vi "Process.vi"(8 "error in":errorcluster, 11 "DAQ_Manager":refnum<class "DAQ_Manager.lvclass">) -> (0 "error out":errorcluster, 3 "DAQ_Manager out":refnum<class "DAQ_Manager.lvclass">)   [LabVIEW 2019, in "DAQ_Manager.lvclass"]
doc: "---------------------------------------------------------------\nJKI State Machine Objects™\nhttp://jki.net/state-machine-objects/\nCopyright (C) 2005-2015, JKI <info@jki.net>\nALL RIGHTS RESERVED"
uses:
  DAQ_Manager.lvclass
  <vilib>/JKI/JKI SMO/SMO/SMO.lvclass
  <vilib>/JKI/JKI SMO/SMO/Typedefs/Parent Call--Enum.ctl
  DAQ/DAQ.lvclass
  DAQ/Typedefs/PublicEvents--DAQ.Read.ctl
  DAQ/Typedefs/PublicEvents--DAQ.Write.ctl
  DAQ/Typedefs/PrivateEvents--DAQ.AI.Channels.ctl
  DAQ/Typedefs/DAQ_Type.ctl
  DAQ/Typedefs/DAQ_SamplingInfo.ctl
  DAQ/Typedefs/DAQ_SamplingMode.ctl
  DAQ/Typedefs/DAQ_Config.ctl
  DAQmx.AO/Typedefs/DAQmx.AO_Config.ctl
  DAQmx.AI/Typedefs/DAQmx.AI_Config.ctl
  DAQmx.AI/Typedefs/AI.Terminal-enum.ctl
  DAQmx.AI/Typedefs/AI.Coupling-enum.ctl
  DAQmx.AO/Typedefs/AO.Terminal-enum.ctl
  Typedefs/PrivateEvents--DAQ_Manager.setDAQConfig.ctl
  C:/Program Files (x86)/National Instruments/LabVIEW 2016/vi.lib/JKI/JKI SMO/SMO/SMO.lvclass
  DAQmx.AI/DAQmx.AI.lvclass
  F:/user/patrick/levy_inst_lockin/src/SMOs/DAQmx/DAQmx.lvclass
  DAQmx.AO/DAQmx.AO.lvclass
  DAQmx/DAQmx.lvclass
  F:/user/patrick/levy_inst_lockin/src/SMOs/DAQ/DAQ.lvclass
  <vilib>/JKI/JKI SMO/SMO/Typedefs/SMOState --Enum.ctl
panel:
  out "DAQ.Read (ms)":u32
  out "DAQ.Read Aggregate (ms)":u32
  out "setWaveform (ms)":u32
  out "Array 2":string[](array[string])
  out "Array":T1[](array[typedef])
  in  "Update Config?":bool
  in  "DAQmx.AO.config":T2[](array[typedef])=[{"output terminal configuration"=-1}] {"output terminal configuration" items=["Default"=-1, "RSE"=10083, "Differential"=10106, "Pseudodifferential"=12529]}
  in  "DAQmx.AI.config":T4[](array[typedef])=[{"AI.Coupling"=10045, "input terminal configuration "=-1}] {"input terminal configuration" items=["default"=-1, "RSE"=10083, "NRSE"=10078, "Differential"=10106, "Pseudodifferential"=12529]; "AI.Coupling" items=["AC"=10045, "DC"=10050, "GND"=10066]}
  in  "DAQ.Config (AO)":T7[](array[typedef])=[{"Channels"="PXI1Slot2/ao0", "DAQ_Type"=enum."AO", "minimum value"=-10.0, "maximum value"=10.0, "DAQ_SamplingInfo"={"Fs"=1000.0, "#s"=1000}, "DAQ_SamplingMode"=enum."Continuous"}] {"maximum value" format="%0.2f"; "minimum value" format="%0.2f"}
  in  "DAQ.Config (AI)":T7[](array[typedef])=[{"Channels"="PXI1Slot2/ai0", "DAQ_Type"=enum."AI", "minimum value"=-10.0, "maximum value"=10.0, "DAQ_SamplingInfo"={"Fs"=1000.0, "#s"=1000}, "DAQ_SamplingMode"=enum."Continuous"}] {"maximum value" format="%0.2f"; "minimum value" format="%0.2f"}
  in  "DAQmx Physical Channels (AO)":tag="PXI1Slot2/ao0:1, PXI1Slot3/ao0:1, PXI1Slot4/ao0:1, PXI1Slot5/ao0:1"
  in  "DAQmx Physical Channels (AI)":tag="PXI1Slot2/ai0:1, PXI1Slot3/ai0:1, PXI1Slot4/ai0:1, PXI1Slot5/ai0:1"
  in  "Simulate?":bool
  # "1. Make a lot of these controls hidden on default Main UI\n    (eg, output terminal)\n2. DAQ.Config etc should be arrays, with each element per device\n3. Make use of most recent lockin controls on front panel\n-- use new enums and arrays per channel/device\n4. DAQ_Manager needs an API for setting the DAQ config (setConfig?)\n5. In process.vi if any Config settings are changed: go to:\nDAQ: stop SMO\nDAQ: init\nDAQ: start SMO\n6. I don't think these need to be controls here in process.vi, they can just be\nchanged through public methods."
  # "DAQ Manager Process.vi"
  # "For instructions on how to use the JKI State Machine Objects, examples and video tutorials, visit:\nhttp://jki.net/state-machine-objects/\n\nJKI State Machine Objects™\nhttp://jki.net/state-machine-objects/\nCopyright (C) 2005-2015, JKI <info@jki.net>\nALL RIGHTS RESERVED"
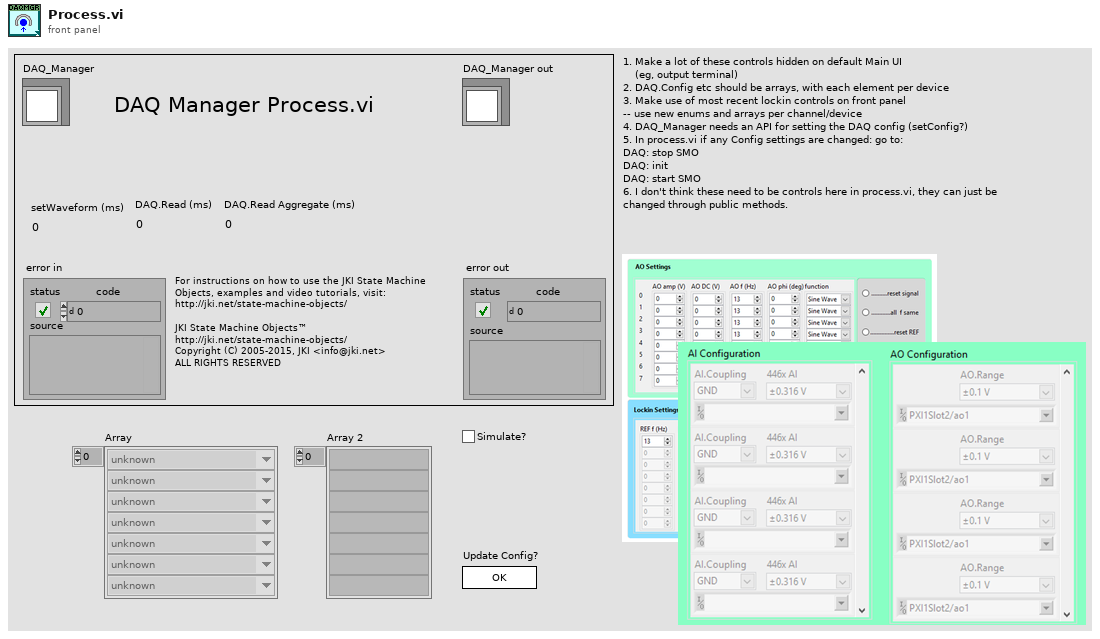
[diagram p1: front panel]
types:
  T1 = typedef "SMO.lvclass/SMOState --Enum.ctl" = enum16{"unknown", "Created", "Started", "Stopped"}
  T2 = typedef "DAQmx.AO.lvclass/DAQmx.AO_Config.ctl" = cluster{"output terminal configuration":T3}
  T3 = typedef "DAQmx.AO.lvclass/AO.Terminal-enum.ctl" = i32
  T4 = typedef "DAQmx.AI.lvclass/DAQmx.AI_Config.ctl" = cluster{"AI.Coupling":T5, "input terminal configuration ":T6}
  T5 = typedef "DAQmx.AI.lvclass/AI.Coupling-enum.ctl" = i32
  T6 = typedef "DAQmx.AI.lvclass/AI.Terminal-enum.ctl" = i32
  T7 = typedef "DAQ.lvclass/DAQ_Config.ctl" = cluster{"Channels":T8, "DAQ_Type":T9, "minimum value":dbl, "maximum value":dbl, "DAQ_SamplingInfo":T10, "DAQ_SamplingMode":T11}
  T8 = typedef "DAQ.lvclass/PrivateEvents--DAQ.AI.Channels.ctl" = string
  T9 = typedef "DAQ.lvclass/DAQ_Type.ctl" = enum16{"AI", "AO"}
  T10 = typedef "DAQ.lvclass/DAQ_SamplingInfo.ctl" = cluster{"Fs":dbl, "#s":i32}
  T11 = typedef "DAQ.lvclass/DAQ_SamplingMode.ctl" = enum16{"Continuous", "Finite"}
  T12 = typedef "SMO.lvclass/Parent Call--Enum.ctl" = enum16{"Allows parent to run", "Does not request parent to run"}
  T13 = typedef "DAQ_Manager.lvclass/PrivateEvents--DAQ_Manager.setDAQConfig.ctl" = cluster{"DAQ.Config (AI)":cluster{"Channels":string, "DAQ_Type":enum16{"AI", "AO"}, "minimum value":dbl, "maximum value":dbl, "DAQ_SamplingInfo":cluster{"Fs":dbl, "#s":i32}, "DAQ_SamplingMode":enum16{"Continuous", "Finite"}}[], "DAQmx.AI.config":T4[], "DAQ.Config (AO)":cluster{"Channels":string, "DAQ_Type":enum16{"AI", "AO"}, "minimum value":dbl, "maximum value":dbl, "DAQ_SamplingInfo":cluster{"Fs":dbl, "#s":i32}, "DAQ_SamplingMode":enum16{"Continuous", "Finite"}}[], "DAQmx.AO.config":T2[]}
  T14 = enum32{"invalid app kind", "Development System", "Run Time System", "Student Edition", "Embedded LabVIEW", "Evaluation", "Custom"}
  T15 = enum32{"Invalid", "Standard", "Closed", "Hidden", "Minimized", "Maximized"}
  T16 = enum32{"Bad", "Idle", "Run top level", "Running"}
  T17 = typedef "DAQ.lvclass/PublicEvents--DAQ.Read.ctl" = waveform(dbl)[]
  T18 = cluster{"Core":cluster{"Current VI Reference":refnum<vi>, "Close Panel on Exit?":bool, "error":errorcluster}, "Self Reference":refnum<class "DAQ_Manager.lvclass">, "Your string data":string, "DAQ":refnum<class "DAQ.lvclass">[], "setWaveform":T17, "to":i32, "AI events":refnum<user-event>[], "DAQ.Config (AO)":T7[], "DAQ.Config (AI)":T7[], "DAQmx.AO.Config":T2[], "DAQmx.AI.Config":T4[]}
  T19 = cluster{"Channels":string, "DAQ_Type":enum16{"AI", "AO"}, "minimum value":dbl, "maximum value":dbl, "DAQ_SamplingInfo":cluster{"Fs":dbl, "#s":i32}, "DAQ_SamplingMode":enum16{"Continuous", "Finite"}}[]
  T20 = typedef "DAQ_Manager.lvclass/PrivateEvents--DAQ_Manager.setWaveform.ctl" = waveform(dbl)[]
  T21 = cluster{"Current VI Reference":refnum<vi>, "Close Panel on Exit?":bool, "error":errorcluster}
  T22 = typedef "SMO.lvclass/Protected Events.ctl" = cluster{"StopProcesses":refnum<user-event>, "AbortProcesses":refnum<user-event>, "Config Changed":refnum<user-event>, "Dependency":refnum<user-event>}
  T23 = typedef "DAQ_Manager.lvclass/PrivateEvents--Cluster.ctl" = cluster{"setWaveform":refnum<user-event>, "setDAQConfig":refnum<user-event>}
  T24 = typedef "DAQ_Manager.lvclass/PublicEvents--Cluster.ctl" = cluster{"getWaveform":refnum<user-event>}
  T25 = typedef "DAQ.lvclass/PublicEvents--Cluster.ctl" = cluster{"DAQ.Read":refnum<user-event>, "DAQ.Write":refnum<user-event>}
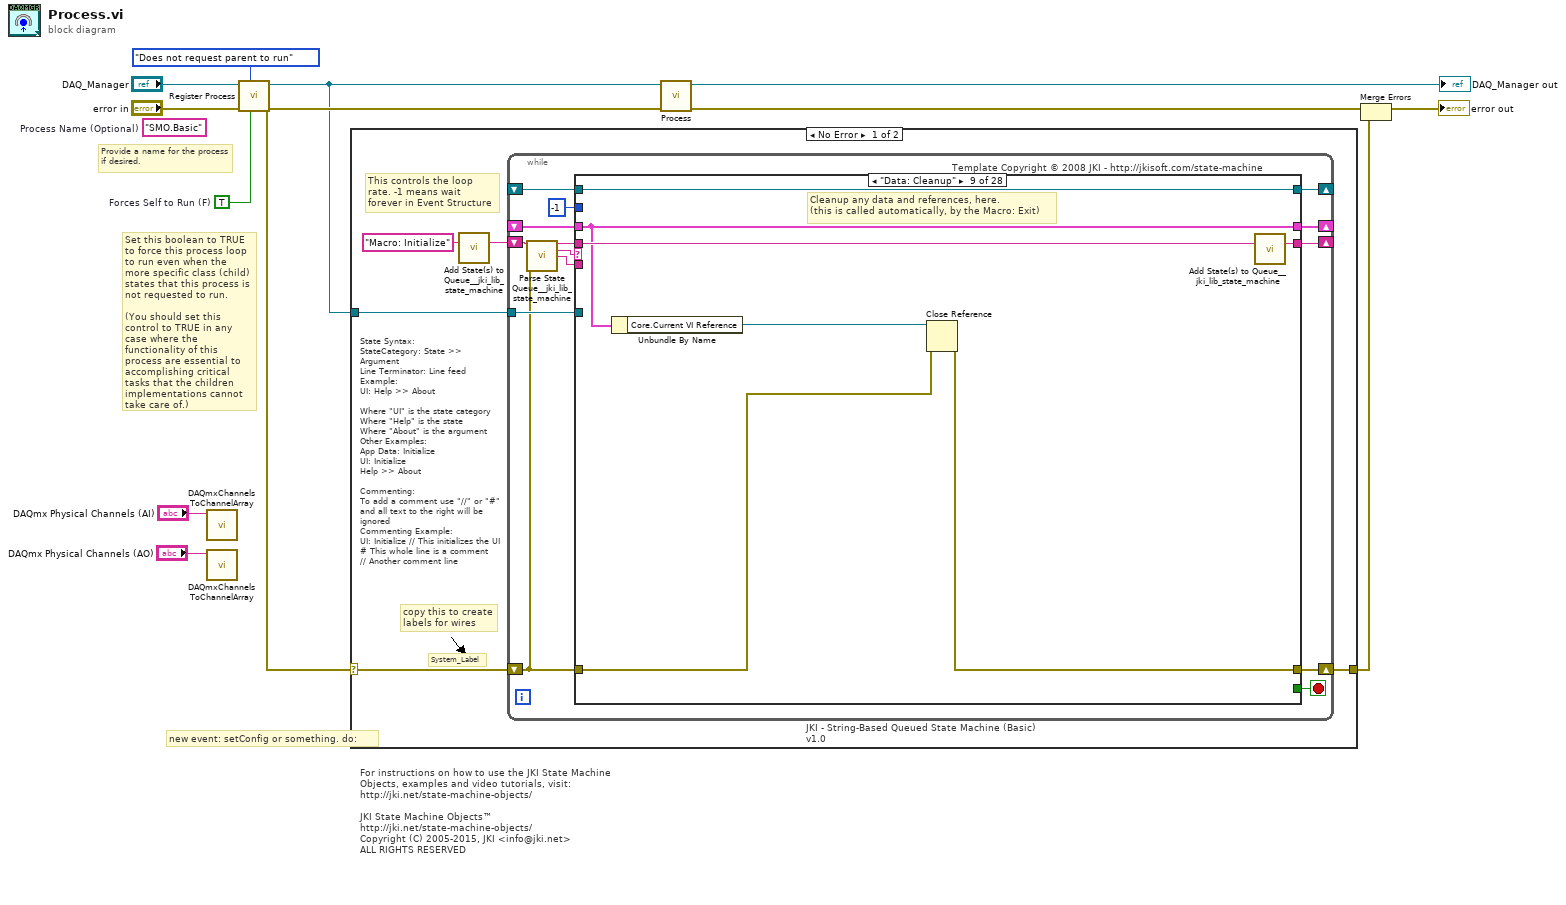
[diagram p0: block diagram]
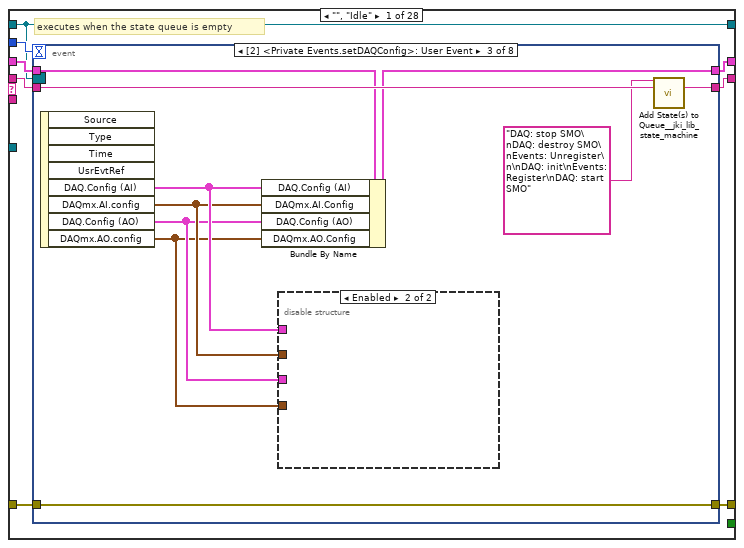
[diagram p2: hidden frame]
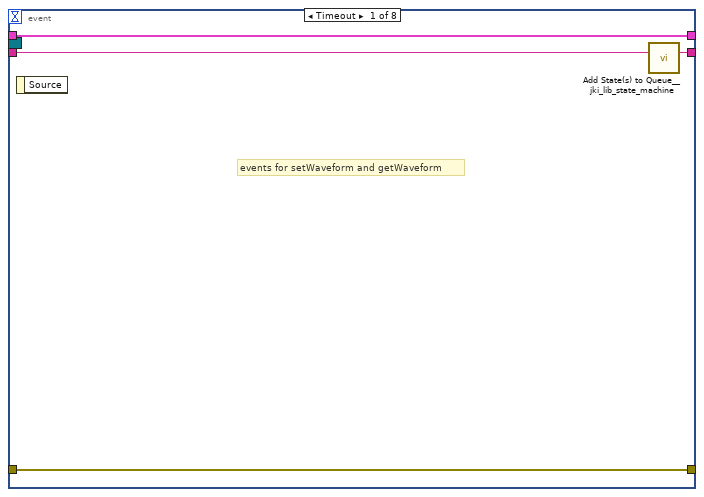
[diagram p3: hidden frame]
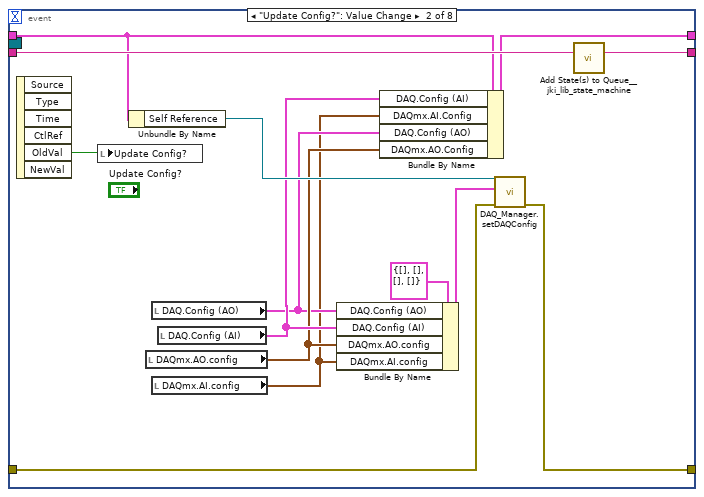
[diagram p4: hidden frame]
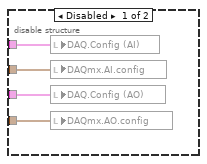
[diagram p5: hidden frame]
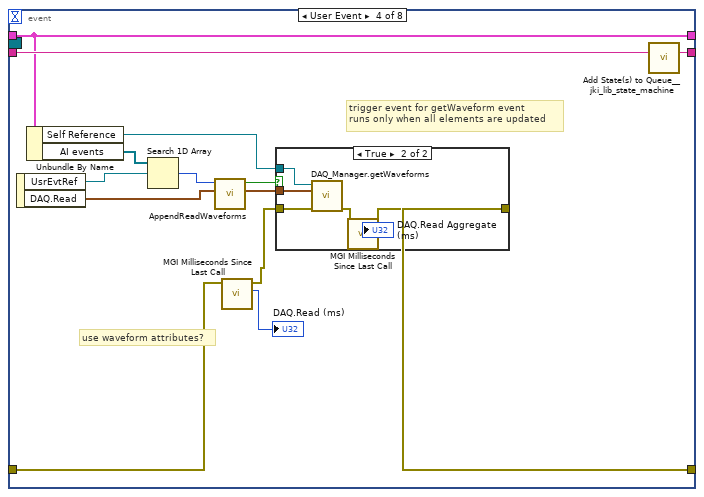
[diagram p6: hidden frame]
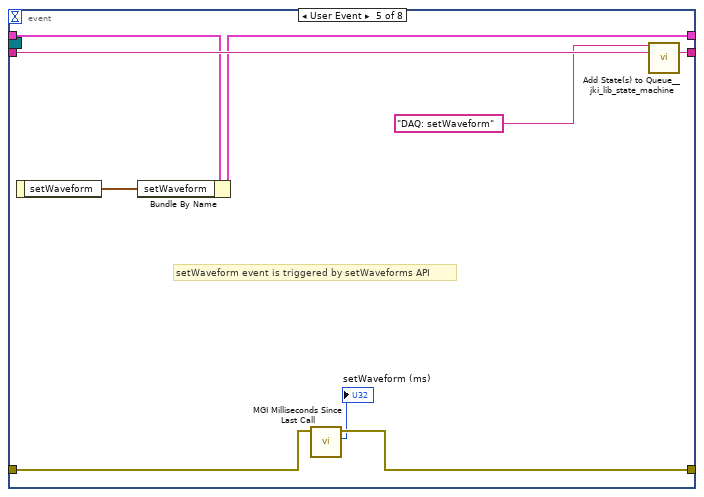
[diagram p8: hidden frame]
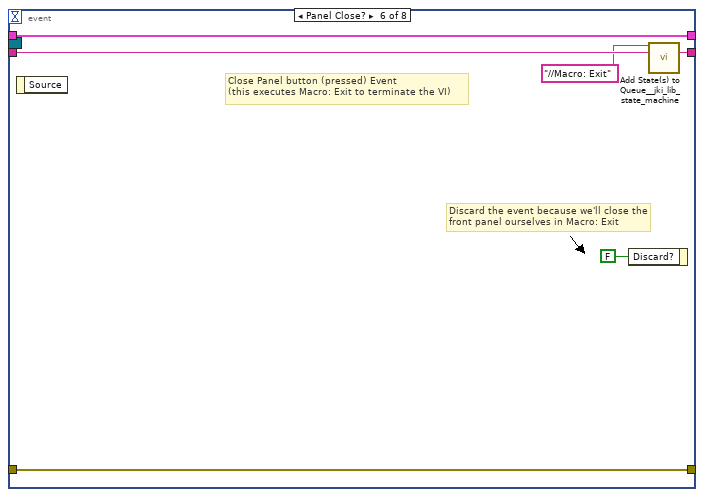
[diagram p9: hidden frame]
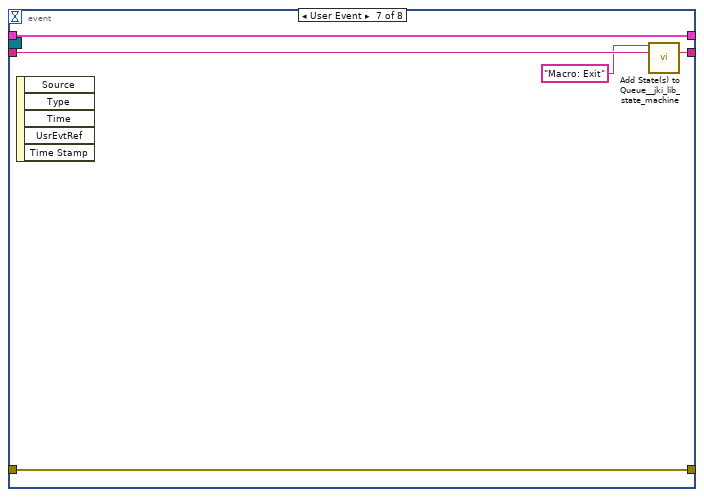
[diagram p10: hidden frame]
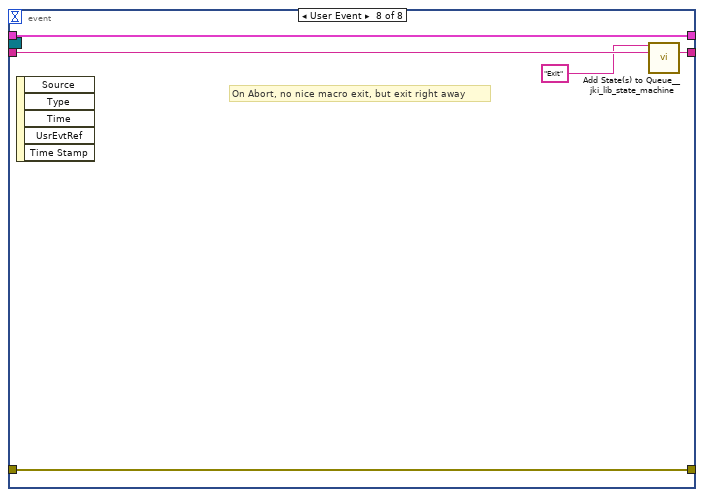
[diagram p11: hidden frame]
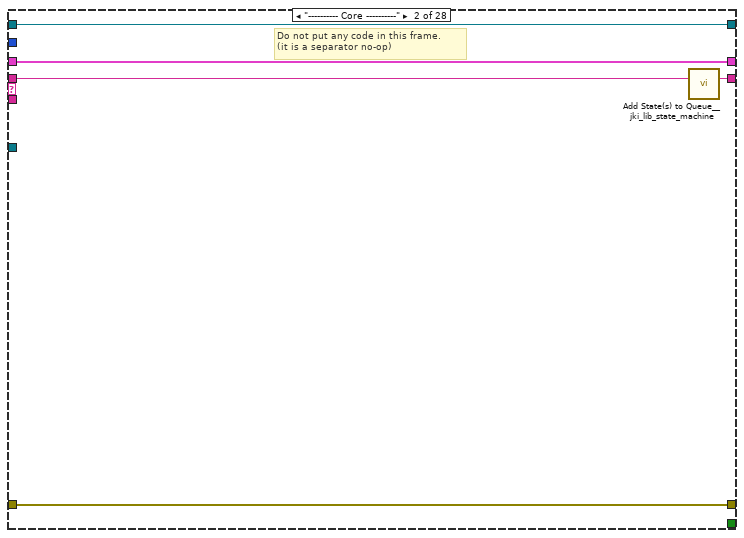
[diagram p12: hidden frame]
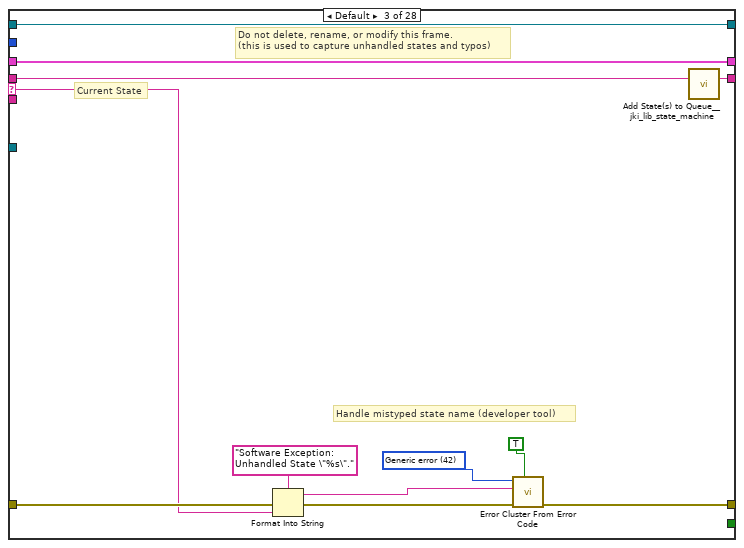
[diagram p13: hidden frame]
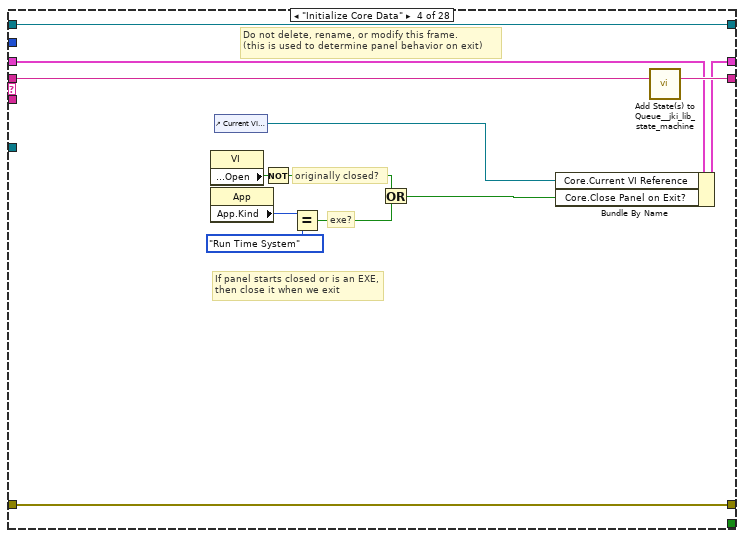
[diagram p14: hidden frame]
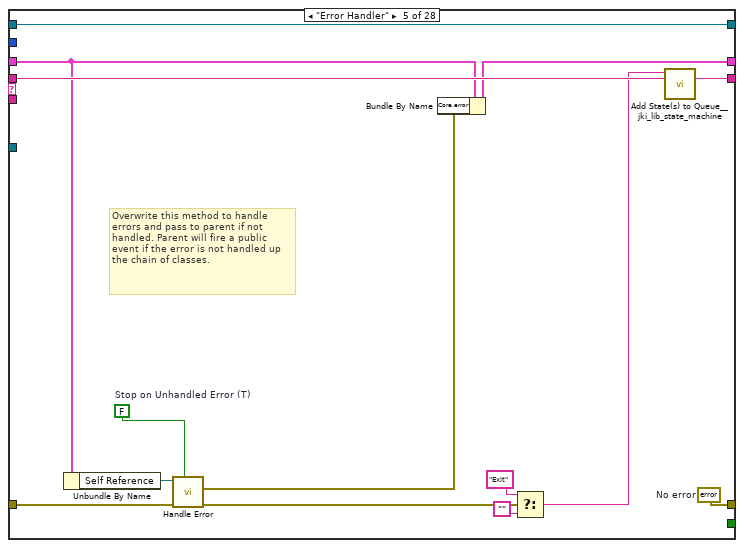
[diagram p15: hidden frame]
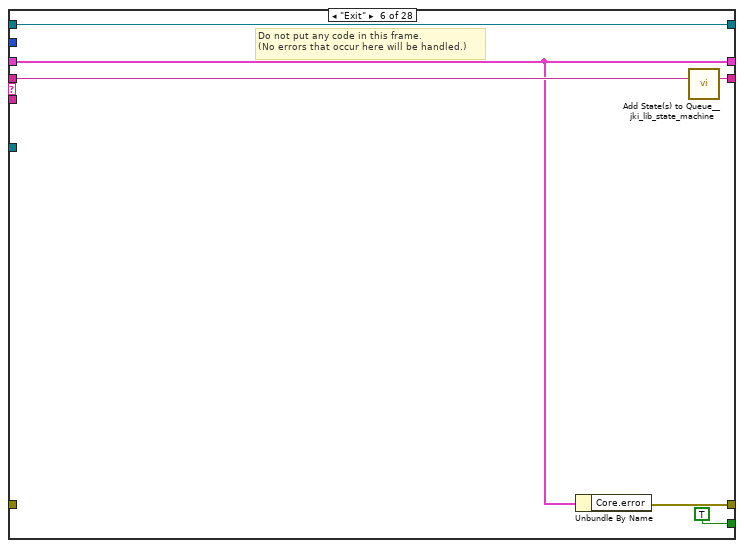
[diagram p16: hidden frame]
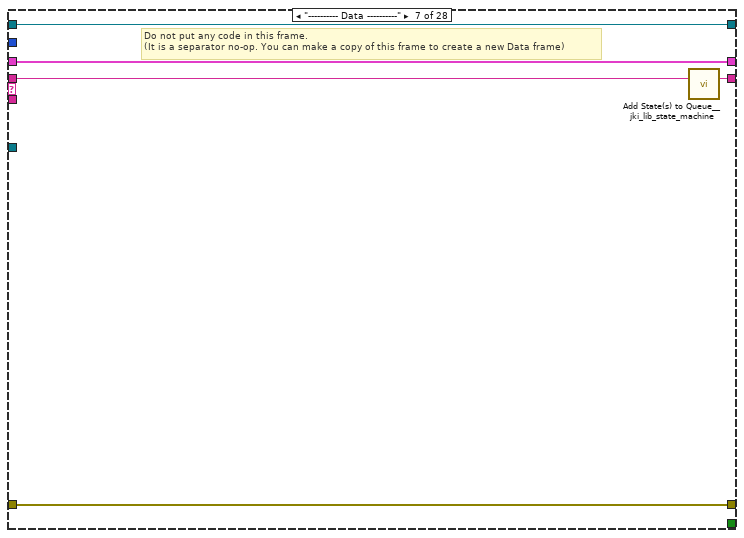
[diagram p17: hidden frame]
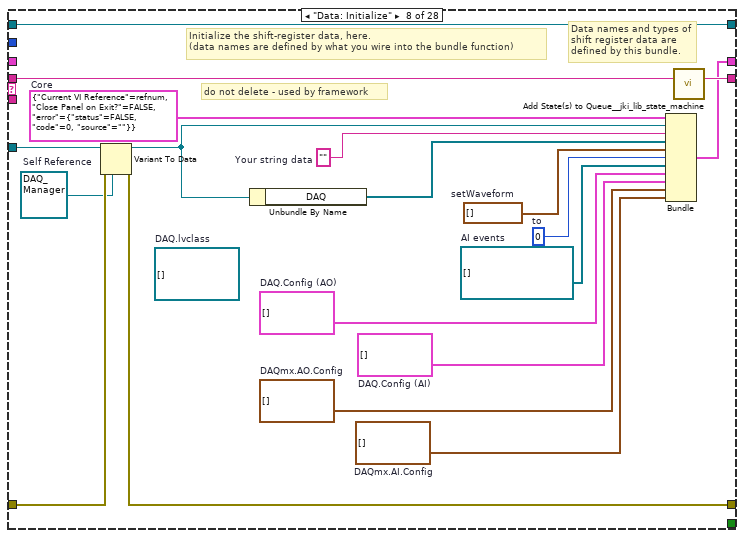
[diagram p18: hidden frame]
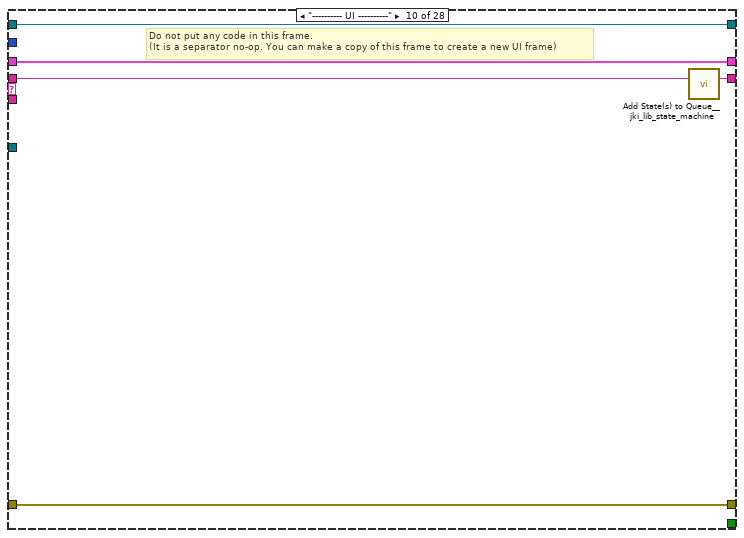
[diagram p19: hidden frame]
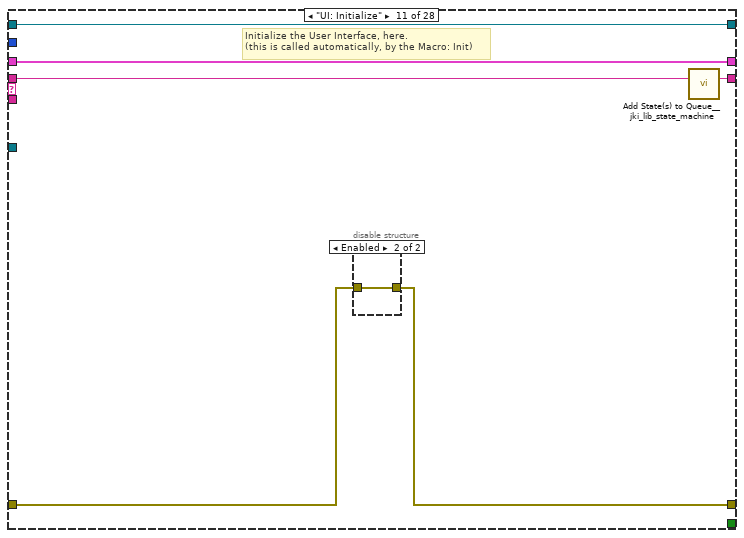
[diagram p20: hidden frame]
diagram:
  w3 = TRUE  # Forces Self to Run (F)
  (unwired) "SMO.Basic"  # Process Name (Optional)
  # "new event: setConfig or something. do:"
  # "Provide a name for the process\nif desired."
  # "Set this boolean to TRUE to force this process loop to run even when the more specific class (child) states that this process is not requested to run.\n\n(You should set this control to TRUE in any case where the functionality of this process are essential to accomplishing critical tasks that the children implementations cannot take care of.)"
  # "For instructions on how to use the JKI State Machine Objects, examples and video tutorials, visit:\nhttp://jki.net/state-machine-objects/\n\nJKI State Machine Objects™\nhttp://jki.net/state-machine-objects/\nCopyright (C) 2005-2015, JKI <info@jki.net>\nALL RIGHTS RESERVED"
  n1 = call "DAQmxChannelsToChannelArray.vi"("DAQmx Physical Channel"="DAQmx Physical Channels (AI)") -> ()  [unwired: 10 in, 1 out]
  n2 = call "DAQmxChannelsToChannelArray.vi"("DAQmx Physical Channel"="DAQmx Physical Channels (AO)") -> ()  [unwired: 10 in, 1 out]
  n3 = call <vilib>:"Register Process.vi"("Forces Self to Run (F)"=w3, "Parent Call"=Parent_Call--Enum."Does not request parent to run", "error in (no error)"="error in", "SMO"="DAQ_Manager") -> ("error out"=w9:errorcluster, "SMO out"=w8:refnum<class "DAQ_Manager.lvclass">)  [unwired: 6 in]
  n4 = case shown="No Error" w9 {
    selector: w9 -> [w14 w492]
    tunnel: w8 -> [w15 _]
    tunnel: [w13 w492] -> w5
    frame No Error {
      # "State Syntax:\nStateCategory: State >> Argument\nLine Terminator: Line feed\nExample:\nUI: Help >> About\n\nWhere \"UI\" is the state category\nWhere \"Help\" is the state\nWhere \"About\" is the argument\nOther Examples:\nApp Data: Initialize\nUI: Initialize\nHelp >> About\n\nCommenting:\nTo add a comment use \"//\" or \"#\" and all text to the right will be ignored\nCommenting Example:\nUI: Initialize // This initializes the UI\n# This whole line is a comment\n// Another comment line"
      # "copy this to create labels for wires"
      # "This controls the loop rate. -1 means wait forever in Event Structure"
      # "System_Label"
      n5 = call <vilib>:"Add State(s) to Queue__jki_lib_state_machine.vi"("State(s) in (\"\")"="Macro: Initialize") -> ("States Out"=w17:string)  [unwired: 14 in]
      n6 = while "JKI - String-Based Queued State Machine (Basic) v1.0" {
        shift-right: [w25] -> _
        shift-left: _ -> [w20]
        shift-right: [w19] -> w13
        shift-left: w14 -> [w21]
        shift-right: [w27] -> _
        shift-left: w17 -> [w28]
        tunnel: w15 -> [w24]
        shift-right: [w23] -> _
        shift-left: _ -> [w22]
        stop <- w26 stop-if-true
        # "Template Copyright © 2008 JKI - http://jkisoft.com/state-machine"
        n7 = call <vilib>:"Parse State Queue__jki_lib_state_machine.vi"("State Queue"=w28, "Error In (no error)"=w21) -> ("Remaining States"=w30:string, "Current State"=w31:string, "Arguments"=w29:string)  [unwired: 11 in]
        n8 = case shown="\"Data: Cleanup\"" w31 {
          selector: w31 -> [_ _ w124 _ _ _ _ _ _ _ _ _ _ _ _ _ _ _ _ _ _ _ _ _ _ _ _ _]
          tunnel: w30 -> [w39 w122 w128 w147 w161 w167 w172 w191 w198 w203 w209 w219 w237 w269 w283 w298 w303 w314 w319 w340 w357 w362 w377 w432 w448 w462 w476 w491]
          tunnel: w29 -> [_ _ _ _ _ _ _ _ _ _ _ w213 w232 _ _ _ _ _ _ _ _ _ _ _ _ _ _ _]
          tunnel: w20 -> [w37 w119 w126 w138 w155 w163 w169 _ w194 w200 w206 w217 w234 w266 w279 w289 w300 w311 w316 w332 w355 w360 w366 w428 w445 w459 w473 w488]
          tunnel: [w38 w121 w127 w146 w160 w166 w171 w190 w197 w202 w208 w218 w236 w268 w282 w297 w302 w313 w318 w339 w356 w361 w376 w431 w447 w461 w475 w490] -> w27
          tunnel: [_ _ _ _ _ TRUE _ _ _ _ _ _ _ _ _ _ _ _ _ _ _ _ _ _ _ _ _ _] -> w26
          tunnel: [w34 w119 w126 w145 w154 w163 w169 w181 w194 w200 w206 w217 w234 w266 w279 w289 w300 w311 w316 w331 w355 w360 w374 w428 w445 w459 w473 w488] -> w25
          tunnel: -1 ("to") -> [w33 _ _ _ _ _ _ _ _ _ _ _ _ _ _ _ _ _ _ _ _ _ _ _ _ _ _ _]
          tunnel: w24 -> [_ _ _ _ _ _ _ w185 _ _ _ _ _ _ _ _ _ _ _ _ _ _ _ _ _ _ _ _]
          tunnel: [w32 w118 w123 w135 w159 w164 w168 w184 w193 w199 w207 w216 w231 w265 w280 w290 w299 w312 w315 w338 w354 w359 w375 w430 w446 w460 w477 w489] -> w23
          tunnel: w22 -> [w32 w118 w123 w135 w159 w164 w168 w184 w193 w199 w207 w216 w231 w265 w280 w290 w299 w312 w315 _ w354 w359 w375 w430 w446 w460 w477 w489]
          tunnel: w21 -> [w35 w120 w129 w144 w157 _ w170 w188 w192 w201 w205 w215 w235 w267 w281 w296 w301 w306 w317 w336 w353 w358 w367 w429 w440 w455 w474 w484]
          tunnel: [w36 w120 w130 w144 w156 w162 w170 w187 w195 w201 w204 w214 w229 w267 w281 w296 w301 w305 w317 w325 w353 w358 w368 w423 w443 w457 w474 w485] -> w19
          frame "", "Idle" {
            # "executes when the state queue is empty"
            n9 = event shown="[2] <Private Events.setDAQConfig>: User Event" {
              selector: w32 -> [_ _ _ _ _ _ _ _]
              dyn-events: _ -> [_ _ _ _ _ _ _ _]
              timeout: w33 -> [_ _ _ _ _ _ _ _]
              tunnel: w39 -> [w43 w56 w66 w85 w101 w107 w112 w117]
              tunnel: [w42 w57 w67 w84 w100 w106 w111 w116] -> w38
              tunnel: w37 -> [w41 w51 w63 w83 w98 w104 w109 w114]
              tunnel: [w40 w44 w64 w77 w94 w105 w110 w115] -> w36
              tunnel: w35 -> [w40 w45 w64 w74 w95 w105 w110 w115]
              tunnel: [w41 w50 w62 w83 w97 w104 w109 w114] -> w34
              event Timeout {
                # "events for setWaveform and getWaveform"
                n10 = event-data() -> ()  [unwired: 1 in, 1 out]
                n11 = call <vilib>:"Add State(s) to Queue__jki_lib_state_machine.vi"("State(s) in (\"\")"=w43) -> ("States Out"=w42:string)  [unwired: 14 in]
              }
              event "Update Config?": Value Change {
                n12 = event-data() -> ("OldVal"=w55:bool)  [unwired: 1 in, 5 out]
                n13 = local write "Update Config?"(w55) -> ()
                n14 = Unbundle By Name(w51) -> ("Self Reference"=w52:refnum<class "DAQ_Manager.lvclass">)
                n15 = local read "DAQmx.AO.config"() -> (w48:T2[])
                n16 = local read "DAQ.Config (AO)"() -> (w47:T7[])
                n17 = local read "DAQmx.AI.config"() -> (w46:T4[])
                n18 = local read "DAQ.Config (AI)"() -> (w49:T7[])
                n19 = Bundle By Name(cluster=T13 {"DAQ.Config (AI)"=[], "DAQmx.AI.config"=[], "DAQ.Config (AO)"=[], "DAQmx.AO.config"=[]} ("DAQ_Manager.setDAQConfig"), "DAQ.Config (AO)"=w47, "DAQ.Config (AI)"=w49, "DAQmx.AO.config"=w48, "DAQmx.AI.config"=w46) -> (w53:T13)
                n20 = Bundle By Name(cluster=w51, "DAQ.Config (AI)"=w49, "DAQmx.AI.Config"=w46, "DAQ.Config (AO)"=w47, "DAQmx.AO.Config"=w48) -> (w50:T18)
                n21 = call "DAQ_Manager.setDAQConfig.vi"("error in (no error)"=w45, "DAQ_Manager.setDAQConfig"=w53, "DAQ_Manager"=w52) -> ("error out"=w44:errorcluster)  [unwired: 7 in, 1 out]
                n22 = call <vilib>:"Add State(s) to Queue__jki_lib_state_machine.vi"("State(s) in (\"\")"=w56) -> ("States Out"=w57:string)  [unwired: 14 in]
              }
              event User Event {
                n23 = event-data() -> ("DAQ.Config (AI)"=w61:T19, "DAQmx.AI.config"=w60:T4[], "DAQ.Config (AO)"=w59:T19, "DAQmx.AO.config"=w58:T2[])  [unwired: 1 in, 4 out]
                n24 = Bundle By Name(cluster=w63, "DAQ.Config (AI)"=w61, "DAQmx.AI.Config"=w60, "DAQ.Config (AO)"=w59, "DAQmx.AO.Config"=w58) -> (w62:T18)
                n25 = disable-structure shown="Enabled" {
                  disable-tunnel: w61 -> [w71 _]
                  disable-tunnel: w60 -> [w70 _]
                  disable-tunnel: w59 -> [w69 _]
                  disable-tunnel: w58 -> [w68 _]
                  frame Disabled {
                    n26 = local write "DAQ.Config (AI)"(w71) -> ()
                    n27 = local write "DAQmx.AI.config"(w70) -> ()
                    n28 = local write "DAQ.Config (AO)"(w69) -> ()
                    n29 = local write "DAQmx.AO.config"(w68) -> ()
                  }
                  frame Enabled {
                  }
                }
                n30 = call <vilib>:"Add State(s) to Queue__jki_lib_state_machine.vi"("State(s) in Front (\"\")"="DAQ: stop SMO\nDAQ: destroy SMO\nEvents: Unregister\n\nDAQ: init\nEvents: Register\nDAQ: start SMO" ("State(s) in Front (\"\")"), "State(s) in (\"\")"=w66) -> ("States Out"=w67:string)  [unwired: 13 in]
              }
              event User Event {
                # "use waveform attributes?"
                # "trigger event for getWaveform event\nruns only when all elements are updated"
                n31 = event-data() -> ("UsrEvtRef"=w81:refnum<user-event>, "DAQ.Read"=w75:waveform(dbl)[])  [unwired: 1 in]
                n32 = Unbundle By Name(w83) -> ("Self Reference"=w78:refnum<class "DAQ_Manager.lvclass">, "AI events"=w82:refnum<user-event>[])
                n33 = Search 1D Array(1D array=w82, element=w81) -> (index of element=w76:i32)  [unwired: 1 in]
                n34 = call "AppendReadWaveforms.vi"("WFM in"=w75, "index of element"=w76) -> ("WFM out"=w80:waveform(dbl)[], "x = y?"=w79:bool)  [unwired: 8 in]
                n35 = call <userlib>:"MGI Milliseconds Since Last Call.vi"("Error In"=w74) -> ("ms"=→"DAQ.Read (ms)":u32, "Error Out"=w73:errorcluster)  [unwired: 5 in]
                n36 = case shown="True" w79 {
                  tunnel: w80 -> [_ w92]
                  tunnel: w78 -> [_ w91]
                  tunnel: w73 -> [w86 w90]
                  tunnel: [w86 w88] -> w77
                  frame False {
                  }
                  frame True {
                    n37 = call "DAQ_Manager.getWaveforms.vi"("error in (no error)"=w90, "getWaveform"=w92, "DAQ_Manager"=w91) -> ("error out"=w89:errorcluster)  [unwired: 7 in, 1 out]
                    n38 = call <userlib>:"MGI Milliseconds Since Last Call.vi"("Error In"=w89) -> ("ms"=→"DAQ.Read Aggregate (ms)":u32, "Error Out"=w88:errorcluster)  [unwired: 5 in]
                  }
                }
                n39 = call <vilib>:"Add State(s) to Queue__jki_lib_state_machine.vi"("State(s) in (\"\")"=w85) -> ("States Out"=w84:string)  [unwired: 14 in]
              }
              event User Event {
                # "setWaveform event is triggered by setWaveforms API"
                n40 = event-data() -> ("setWaveform"=w99:T20)  [unwired: 1 in]
                n41 = Bundle By Name(cluster=w98, "setWaveform"=w99) -> (w97:T18)
                n42 = call <userlib>:"MGI Milliseconds Since Last Call.vi"("Error In"=w95) -> ("ms"=→"setWaveform (ms)":u32, "Error Out"=w94:errorcluster)  [unwired: 5 in]
                n43 = call <vilib>:"Add State(s) to Queue__jki_lib_state_machine.vi"("State(s) in Front (\"\")"="DAQ: setWaveform" ("State(s) in Front (\"\")"), "State(s) in (\"\")"=w101) -> ("States Out"=w100:string)  [unwired: 13 in]
              }
              event Panel Close? {
                # "Discard the event because we'll close the front panel ourselves in Macro: Exit"
                # "Close Panel button (pressed) Event\n(this executes Macro: Exit to terminate the VI)"
                n44 = event-data() -> ()  [unwired: 1 in, 1 out]
                n45 = event-data("Discard?"=FALSE) -> ()  [unwired: 1 in, 1 out]
                n46 = call <vilib>:"Add State(s) to Queue__jki_lib_state_machine.vi"("State(s) in Front (\"\")"="//Macro: Exit", "State(s) in (\"\")"=w107) -> ("States Out"=w106:string)  [unwired: 13 in]
              }
              event User Event {
                n47 = event-data() -> ()  [unwired: 1 in, 5 out]
                n48 = call <vilib>:"Add State(s) to Queue__jki_lib_state_machine.vi"("State(s) in Front (\"\")"="Macro: Exit", "State(s) in (\"\")"=w112) -> ("States Out"=w111:string)  [unwired: 13 in]
              }
              event User Event {
                # "On Abort, no nice macro exit, but exit right away"
                n49 = event-data() -> ()  [unwired: 1 in, 5 out]
                n50 = call <vilib>:"Add State(s) to Queue__jki_lib_state_machine.vi"("State(s) in Front (\"\")"="Exit", "State(s) in (\"\")"=w117) -> ("States Out"=w116:string)  [unwired: 13 in]
              }
            }
          }
          frame "---------- Core ----------" {
            # "Do not put any code in this frame.\n(it is a separator no-op)"
            n51 = call <vilib>:"Add State(s) to Queue__jki_lib_state_machine.vi"("State(s) in (\"\")"=w122) -> ("States Out"=w121:string)  [unwired: 14 in]
          }
          frame Default {
            w133 = 42 items=["No error", "Argument error", "Memory is full", "Out of zone", "End of file", "File already open", "Generic file I/O error", "File not found", "File permission error", "Disk is full", "Duplicate path", "Too many files open", "System feature not enabled", "Resource file not found", "Cannot add resource", "Resource not found", "Image not found", "Image memory error", "Pen does not exist", "Config type invalid", "Config token not found", "Config parse error", "Config memory error", "Bad external code format", "Bad external code offset", "External code not present", "Null window", "Destroy window error", "Null menu", "Print aborted", "Bad print record", "Print driver error", "Windows error during printing", "Memory error during printing", "Print dialog error", "Generic print error", "Invalid device refnum", "Device not found", "Device parameter error", "Device unit error", "Cannot open device", "Device call aborted", "Generic error", "Cancelled by user", "Object ID too low", "Object ID too high", "Object not in heap", "Unknown heap", "Unknown object (invalid DefProc)", "Unknown object (DefProc not in table)", "Message out of range", "Invalid (null) method", "Unknown message", "Manager call not supported", "Bad address", "Network operation in progress", "Network operation timed out", "Connection is busy", "Network attribute not supported", "Network error", "Address in use", "System out of memory", "Connection aborted", "Connection refused", "Not connected", "Already connected", "Connection closed", "Initialization error (interapplication manager)", "Bad occurrence", "Wait on unbound occurrence handler", "Occurrence queue overflow", "Datalog type conflict", "Unused", "Unrecognized type (interapplication manager)", "Memory corrupt", "Failed to make temporary DLL", "Old CIN version", "Drag socket not found", "Failed to load drop-object", "Failed to register OLE object", "Failed to release OLE object", "Format specifier type mismatch", "Unknown format specifier", "Too few format specifiers", "Too many format specifiers", "Scan failed", "Newer CIN version", "Error converting to variant", "Runtime menu error", "Password tampered", "Variant attribute not found", "Incompatible variant data type", "Event data is not available", "Event Store is not present", "Occurrence is not found", "Event Queue is not created", "Event info is not available", "Refnum passed is NULL", "Error retrieving Class GUID", "Error retrieving CoClass GUID", "Error retrieving TypeLib GUID.", "Bad built application magic bytes.", "Specific driver is different from the specific driver associated with the Logical Name.", "There is no session opened to the class driver.", "Max Error", "MAX - Error with config objects", "MAX - Error loading configuration", "MAX - Group not supported"]
            # "Current State"
            # "Do not delete, rename, or modify this frame.\n(this is used to capture unhandled states and typos)"
            # "Handle mistyped state name (developer tool)"
            n52 = Format Into String(format string="Software Exception: Unhandled State \"%s\"." ("message"), error in=w129, w124) -> (resulting string=w132:string, error out=w131:errorcluster)  [unwired: 1 in]
            n53 = call <vilib>:"Error Cluster From Error Code.vi"("show call chain? (False)"=TRUE, "error in (no error)"=w131, "error message (\"\")"=w132, "error code (0)"=w133) -> ("error out"=w130:errorcluster)  [unwired: 5 in]
            n54 = call <vilib>:"Add State(s) to Queue__jki_lib_state_machine.vi"("State(s) in (\"\")"=w128) -> ("States Out"=w127:string)  [unwired: 14 in]
          }
          frame "Initialize Core Data" {
            # "Do not delete, rename, or modify this frame.\n(this is used to determine panel behavior on exit)"
            # "originally closed?"
            # "exe?"
            # "If panel starts closed or is an EXE, then close it when we exit"
            n55 = property class="VI"() -> ("Front Panel.Open"=w143:bool)  [unwired: 2 in, 2 out]
            n56 = property class="App"() -> ("App.Kind"=w142:T14)  [unwired: 2 in, 2 out]
            n57 = control-ref of="Current VI Reference"() -> (w136:refnum<vi>)
            n58 = Not(x=w143) -> (.not. x?=w140:bool)
            n59 = Equal?(x=w142, y=T14."Run Time System" ("Application:Kind")) -> (x = y?=w139:bool)
            n60 = Or(x=w140, y=w139) -> (x .or. y?=w137:bool)
            n61 = Bundle By Name(cluster=w138, "Core.Current VI Reference"=w136, "Core.Close Panel on Exit?"=w137) -> (w145:T18)
            n62 = call <vilib>:"Add State(s) to Queue__jki_lib_state_machine.vi"("State(s) in (\"\")"=w147) -> ("States Out"=w146:string)  [unwired: 14 in]
          }
          frame "Error Handler" {
            w148 = FALSE  # Stop on Unhandled Error (T)
            w156 = errorcluster {"status"=FALSE, "code"=0, "source"=""}  # No error
            # "Overwrite this method to handle errors and pass to parent if not handled. Parent will fire a public event if the error is not handled up the chain of classes."
            n63 = Unbundle By Name(w155) -> ("Self Reference"=w158:refnum<class "DAQ_Manager.lvclass">)
            n64 = call-dynamic "Handle Error.vi"("Stop on Unhandled Error (T)"=w148, "error in"=w157, "SMO"=w158) -> ("handling error"=w149:errorcluster, "Unhandled error"=w152:errorcluster)  [unwired: 6 in, 1 out]
            n65 = Bundle By Name(cluster=w155, "Core.error"=w152) -> (w154:T18)
            n66 = Select(t="Exit", s=w149, f="") -> (s? t:f=w153:string)
            n67 = call <vilib>:"Add State(s) to Queue__jki_lib_state_machine.vi"("State(s) in Front (\"\")"=w153, "State(s) in (\"\")"=w161) -> ("States Out"=w160:string)  [unwired: 13 in]
          }
          frame "Exit" {
            # "Do not put any code in this frame.\n(No errors that occur here will be handled.)"
            n68 = Unbundle By Name(w163) -> ("Core.error"=w162:errorcluster)
            n69 = call <vilib>:"Add State(s) to Queue__jki_lib_state_machine.vi"("State(s) in (\"\")"=w167) -> ("States Out"=w166:string)  [unwired: 14 in]
          }
          frame "---------- Data ----------" {
            # "Do not put any code in this frame.\n(It is a separator no-op. You can make a copy of this frame to create a new Data frame)"
            n70 = call <vilib>:"Add State(s) to Queue__jki_lib_state_machine.vi"("State(s) in (\"\")"=w172) -> ("States Out"=w171:string)  [unwired: 14 in]
          }
          frame "Data: Initialize" {
            w175 = T4[] []  # DAQmx.AI.Config
            w176 = T2[] []  # DAQmx.AO.Config
            w177 = T7[] []  # DAQ.Config (AI)
            w178 = T7[] []  # DAQ.Config (AO)
            w179 = refnum<user-event>[] []  # AI events
            w180 = T17 []  # setWaveform
            w182 = 0  # to
            (unwired) refnum<class "DAQ.lvclass">[] []  # DAQ.lvclass
            w183 = T21 {"Current VI Reference"=refnum, "Close Panel on Exit?"=FALSE, "error"={"status"=FALSE, "code"=0, "source"=""}}  # Core
            w186 = refnum<class "DAQ_Manager.lvclass"> refnum  # Self Reference
            w189 = ""  # Your string data
            # "do not delete - used by framework"
            # "Data names and types of shift register data are defined by this bundle."
            # "Initialize the shift-register data, here.\n(data names are defined by what you wire into the bundle function)"
            n71 = Variant To Data(error in=w188, type=w186, Variant=w185) -> (data=w174:refnum<class "DAQ_Manager.lvclass">, error out=w187:errorcluster)
            n72 = Unbundle By Name(w174) -> ("DAQ"=w173:refnum<class "DAQ.lvclass">[])
            n73 = Bundle("Core"=w183, "Self Reference"=w174, "Your string data"=w189, "DAQ"=w173, "setWaveform"=w180, "to"=w182, "AI events"=w179, "DAQ.Config (AO)"=w178, "DAQ.Config (AI)"=w177, "DAQmx.AO.Config"=w176, "DAQmx.AI.Config"=w175) -> (w181:T18)  [unwired: 1 in]
            n74 = call <vilib>:"Add State(s) to Queue__jki_lib_state_machine.vi"("State(s) in (\"\")"=w191) -> ("States Out"=w190:string)  [unwired: 14 in]
          }
          frame "Data: Cleanup" {
            # "Cleanup any data and references, here.\n(this is called automatically, by the Macro: Exit)"
            n75 = Unbundle By Name(w194) -> ("Core.Current VI Reference"=w196:refnum<vi>)
            n76 = Close Reference(reference=w196, error in (no error)=w192) -> (error out=w195:errorcluster)
            n77 = call <vilib>:"Add State(s) to Queue__jki_lib_state_machine.vi"("State(s) in (\"\")"=w198) -> ("States Out"=w197:string)  [unwired: 14 in]
          }
          frame "---------- UI ----------" {
            # "Do not put any code in this frame.\n(It is a separator no-op. You can make a copy of this frame to create a new UI frame)"
            n78 = call <vilib>:"Add State(s) to Queue__jki_lib_state_machine.vi"("State(s) in (\"\")"=w203) -> ("States Out"=w202:string)  [unwired: 14 in]
          }
          frame "UI: Initialize" {
            # "Initialize the User Interface, here.\n(this is called automatically, by the Macro: Init)"
            n79 = disable-structure shown="Enabled" {
              disable-tunnel: w205 -> [w211 w212]
              disable-tunnel: [w210 w212] -> w204
              frame Disabled {
                n80 = call <userlib>:"Fit VI window to Largest Dec__ogtk.vi"("error in (no error)"=w211) -> ("error out"=w210:errorcluster)  [unwired: 5 in, 1 out]
              }
              frame Enabled {
              }
            }
            n81 = call <vilib>:"Add State(s) to Queue__jki_lib_state_machine.vi"("State(s) in (\"\")"=w209) -> ("States Out"=w208:string)  [unwired: 14 in]
          }
          frame "UI: Cursor Set" {
            # "Argument"
            # "Initialize the User Interface, here.\n(this is called automatically, by the Macro: Init)"
            n82 = disable-structure shown="Default" {
              disable-tunnel: w215 -> [w220 w223]
              disable-tunnel: [w220 w222] -> w214
              disable-tunnel: w213 -> [_ w221]
              frame condition #0 {
              }
              frame condition #1 (active) {
                n83 = case shown="\"Idle\", Default" w221 {
                  tunnel: w223 -> [w225 w227]
                  tunnel: [w224 w226] -> w222
                  frame "Idle", Default {
                    n84 = call <vilib>:"Unset Busy.vi"("error in (no error)"=w225) -> ("error out"=w224:errorcluster)  [unwired: 10 in]
                  }
                  frame "Busy" {
                    n85 = call <vilib>:"Set Busy.vi"("error in (no error)"=w227) -> ("error out"=w226:errorcluster)  [unwired: 9 in, 1 out]
                  }
                }
              }
            }
            n86 = call <vilib>:"Add State(s) to Queue__jki_lib_state_machine.vi"("State(s) in (\"\")"=w219) -> ("States Out"=w218:string)  [unwired: 14 in]
          }
          frame "UI: Front Panel State" {
            # "use for debugging"
            # "Argument"
            # "Set Front Panel Open or Closed\n(Usage: \"UI: Front Panel State >> Open|Close\")"
            n87 = Unbundle By Name(w234) -> ("Core.Current VI Reference"=w233:refnum<vi>)
            n88 = disable-structure shown="Default" {
              disable-tunnel: w235 -> [w241 w264]
              disable-tunnel: [w240 w264] -> w230
              disable-tunnel: w233 -> [w239 _]
              disable-tunnel: w232 -> [w238 _]
              frame condition #0 (active) {
                n89 = case shown="\"Close\"" w238 {
                  tunnel: w241 -> [w245 w258]
                  tunnel: [w247 w259] -> w240
                  tunnel: w239 -> [w246 w256]
                  frame "Open", Default {
                    n90 = property class="VI"(reference=w246, error in=w245) -> (reference out=w243:refnum<vi>, error out=w244:errorcluster, "FP.State"=w242:T15)
                    n91 = case shown="\"Closed\"" w242 {
                      tunnel: [w250 w253] -> w247
                      tunnel: w244 -> [w249 w253]
                      tunnel: w243 -> [w248 _]
                      frame "Closed" {
                        n92 = invoke class="VI" method="FP.Open"(reference=w248, error in=w249, "Activate"=TRUE, "State"=T15."Standard") -> (error out=w250:errorcluster)  [unwired: 1 in, 4 out]
                      }
                      frame Default {
                      }
                    }
                  }
                  frame "Close" {
                    n93 = property class="VI"(reference=w256, error in=w258) -> (reference out=w255:refnum<vi>, error out=w257:errorcluster, "FP.State"=w254:T15)
                    n94 = case shown="Default" w254 {
                      tunnel: [w260 w263] -> w259
                      tunnel: w257 -> [w260 w262]
                      tunnel: w255 -> [_ w261]
                      frame "Invalid", "Closed" {
                      }
                      frame Default {
                        n95 = invoke class="VI" method="FP.Close"(reference=w261, error in=w262) -> (error out=w263:errorcluster)  [unwired: 1 in, 2 out]
                      }
                    }
                  }
                }
              }
              frame condition #1 {
              }
            }
            n96 = call <userlib>:"Wait (ms)__ogtk.vi"("error in (no error)"=w230, "milliseconds to wait"=u32 0) -> ("error out"=w229:errorcluster)  [unwired: 8 in, 1 out]
            n97 = call <vilib>:"Add State(s) to Queue__jki_lib_state_machine.vi"("State(s) in (\"\")"=w237) -> ("States Out"=w236:string)  [unwired: 14 in]
          }
          frame "---------- Macro ----------" {
            # "Do not put any code in this frame.\n(It is a separator no-op. You can make a copy of this frame to create a new Macro frame)"
            n98 = call <vilib>:"Add State(s) to Queue__jki_lib_state_machine.vi"("State(s) in (\"\")"=w269) -> ("States Out"=w268:string)  [unwired: 14 in]
          }
          frame "Macro: Initialize" {
            w270 = "Process: Sync"
            # "Initialization Macro\n(This is called once, when the VI starts)"
            n99 = control-ref of="This VI"() -> (w272:refnum<vi>)
            n100 = property class="VI"(reference=w272) -> ("Exec.State"=w271:T16)  [unwired: 1 in, 2 out]
            n101 = Equal?(x=w271, y=T16."Run top level") -> (x = y?=w277:bool)
            n102 = Select(t=w270, s=w277, f="") -> ()  [unwired: 1 out]
            n103 = call <vilib>:"Add State(s) to Queue__jki_lib_state_machine.vi"("State(s) in Front (\"\")"="Data: Initialize\nInitialize Core Data\nUI: Initialize\nUI: Front Panel State >> Open\n//DAQ: update config\nEvents: Register\n//DAQ: init", "State(s) in (\"\")"=w270, "State(s) at Back (\"\")"="//DAQ: start SMO") -> ("States Out"=w273:string)  [unwired: 12 in]
            n104 = call <vilib>:"Add State(s) to Queue__jki_lib_state_machine.vi"("State(s) in Front (\"\")"=w273, "State(s) in (\"\")"=w283) -> ("States Out"=w282:string)  [unwired: 13 in]
          }
          frame "Macro: Exit" {
            # "Exit Macro\n(This is called once, when the VI exits)"
            n105 = Unbundle By Name(w289) -> ("Core.Close Panel on Exit?"=w295:bool)
            n106 = Select(t="UI: Front Panel State >> Open", s=w295, f="") -> (s? t:f=w292:string)
            n107 = call <vilib>:"Add State(s) to Queue__jki_lib_state_machine.vi"("State(s) in Front (\"\")"="Data: Cleanup\nEvents: Unregister", "State(s) in (\"\")"="Process: Sync", "State(s) at Back (\"\")"="Exit") -> ("States Out"=w286:string)  [unwired: 12 in]
            n108 = call <vilib>:"Add State(s) to Queue__jki_lib_state_machine.vi"("State(s) in Front (\"\")"="DAQ: stop SMO\nDAQ: destroy SMO", "State(s) in (\"\")"=w292, "State(s) at Back (\"\")"=w286) -> ("States Out"=w291:string)  [unwired: 12 in]
            n109 = call <vilib>:"Add State(s) to Queue__jki_lib_state_machine.vi"("State(s) in Front (\"\")"=w291, "State(s) in (\"\")"=w298) -> ("States Out"=w297:string)  [unwired: 13 in]
          }
          frame "---------- Process ----------" {
            # "Template Separator\n(You can make a copy of, or modify, this frame)"
            n110 = call <vilib>:"Add State(s) to Queue__jki_lib_state_machine.vi"("State(s) in (\"\")"=w303) -> ("States Out"=w302:string)  [unwired: 14 in]
          }
          frame "Process: Sync" {
            n111 = Unbundle By Name(w311) -> ("Self Reference"=w307:refnum<class "DAQ_Manager.lvclass">)
            n112 = call <vilib>:"WaitOnProcessSync.vi"("error in (no error)"=w306, "SMO"=w307) -> ("error out"=w305:errorcluster, "Don't run?"=w310:bool)  [unwired: 7 in, 1 out]
            n113 = Select(t="Data: Cleanup\nEvents: Unregister\nExit", s=w310, f="") -> (s? t:f=w304:string)
            n114 = call <vilib>:"Add State(s) to Queue__jki_lib_state_machine.vi"("State(s) in Front (\"\")"=w304, "State(s) in (\"\")"=w314) -> ("States Out"=w313:string)  [unwired: 13 in]
          }
          frame "---------- Events ----------" {
            # "Template Separator\n(You can make a copy of, or modify, this frame)"
            n115 = call <vilib>:"Add State(s) to Queue__jki_lib_state_machine.vi"("State(s) in (\"\")"=w319) -> ("States Out"=w318:string)  [unwired: 14 in]
          }
          frame "Events: Register" {
            # "GetPublicEvents of DAQManager"
            # "GetPublicEvents of DAQ"
            # "GetPrivateEvents of DAQManager"
            n116 = Unbundle By Name(w332) -> ("Self Reference"=w337:refnum<class "DAQ_Manager.lvclass">)
            n117 = call <vilib>:"GetProtectedEvents.vi"("error in (no error)"=w336, "SMO"=w337) -> ("error out"=w320:errorcluster, "SMO Protected Events"=w334:T22, "SMO out"=w330:refnum<class "DAQ_Manager.lvclass">)  [unwired: 7 in]
            n118 = Unbundle By Name(w332) -> ("DAQ"=w327:refnum<class "DAQ.lvclass">[])
            n119 = call "DAQ_Manager.GetPrivateEvents.vi"("DAQ_Manager"=w330) -> ("error out"=w321:errorcluster, "Private Events"=w335:T23, "DAQ_Manager out"=w328:refnum<class "DAQ_Manager.lvclass">)  [unwired: 8 in]
            n120 = call "DAQ_Manager.GetPublicEvents.vi"("DAQ_Manager"=w328) -> ("error out"=w322:errorcluster, "DAQManager.Public Events"=w329:T24)  [unwired: 8 in, 1 out]
            n121 = for {
              tunnel: w327 -> [w347] mode=indexing
              shift-right: [w351] -> w323
              shift-left: _ -> [w345]
              tunnel: [w349] -> w333 mode=indexing if=w341
              n122 = call "getDAQ_Config.vi"("error in (no error)"=w345, "DAQ in"=w347) -> ("error out"=w346:errorcluster, "DAQ_Config"=w344:T7, "DAQ out"=w348:refnum<class "DAQ.lvclass">)  [unwired: 7 in]
              n123 = call "DAQ.GetPublicEvents.vi"("error in (no error)"=w346, "DAQ"=w348) -> ("error out"=w351:errorcluster, "Public Events"=w350:T25)  [unwired: 7 in, 1 out]
              n124 = Unbundle By Name(w344) -> ("DAQ_Type"=w343:T9)
              n125 = Unbundle By Name(w350) -> ("DAQ.Read"=w349:refnum<user-event>)
              n126 = Equal?(x=DAQ_Type."AI" ("DAQ_Type"), y=w343) -> (x = y?=w341:bool)
            }
            n127 = call "RenameReadEvents.vi"("DAQ.Read"=w333) -> ("DAQ.Read"=w326:refnum<user-event>[])
            n128 = register-events(w334, w335, w329, w326) -> (reference out=w338:refnum<event-registration>, error out=w324:errorcluster)  [unwired: 2 in]
            n129 = Bundle By Name(cluster=w332, "AI events"=w326) -> (w331:T18)
            n130 = Merge Errors(w320, w324, w323, w322, w321) -> (w325:errorcluster)
            n131 = call <vilib>:"Add State(s) to Queue__jki_lib_state_machine.vi"("State(s) in (\"\")"=w340) -> ("States Out"=w339:string)  [unwired: 14 in]
          }
          frame "Events: Unregister" {
            n132 = Unregister For Events(event registration refnum=w354, error in=w353) -> (error out=w352:errorcluster)
            n133 = call <vilib>:"Clear Errors.vi"("error in (no error)"=w352) -> ()  [unwired: 5 in, 2 out]
            n134 = call <vilib>:"Add State(s) to Queue__jki_lib_state_machine.vi"("State(s) in (\"\")"=w357) -> ("States Out"=w356:string)  [unwired: 14 in]
          }
          frame "---------- DAQ ----------" {
            n135 = call <vilib>:"Add State(s) to Queue__jki_lib_state_machine.vi"("State(s) in (\"\")"=w362) -> ("States Out"=w361:string)  [unwired: 14 in]
          }
          frame "DAQ: init" {
            # "I don't think TO is relevant here. More important for DAQ SMO?"
            n136 = Unbundle By Name(w366) -> ("DAQ.Config (AI)"=w372:T7[], "DAQmx.AI.Config"=w369:T4[], "DAQ.Config (AO)"=w371:T7[], "DAQmx.AO.Config"=w370:T2[])
            n137 = case shown="False" "Simulate?" {
              tunnel: w371 -> [w395 w414]
              tunnel: w370 -> [w394 _]
              tunnel: w372 -> [w393 w413]
              tunnel: w369 -> [w392 _]
              tunnel: [w387 w407] -> w368
              tunnel: [w386 w408] -> w363
              tunnel: w367 -> [w383 w406]
              frame False {
                n138 = for {
                  tunnel: w395 -> [w400] mode=indexing
                  tunnel: w394 -> [w399] mode=indexing
                  tunnel: [w398] -> w390 mode=indexing
                  shift-right: [w397] -> w388
                  shift-left: w383 -> [w396]
                  n139 = call "createDAQmx.AO.vi"("error in (no error)"=w396, "DAQmx.AO.config"=w399, "DAQ.Config"=w400) -> ("error out"=w397:errorcluster, "DAQmx.AO out"=w398:refnum<class "DAQmx.AO.lvclass">)  [unwired: 7 in]
                }
                n140 = for {
                  tunnel: w393 -> [w405] mode=indexing
                  tunnel: w392 -> [w404] mode=indexing
                  tunnel: [w402] -> w391 mode=indexing
                  shift-right: [w403] -> w389
                  shift-left: w383 -> [w401]
                  n141 = call "createDAQmx.AI.vi"("error in (no error)"=w401, "DAQmx.AI.config"=w404, "DAQ.config"=w405) -> ("error out"=w403:errorcluster, "DAQmx.AI out"=w402:refnum<class "DAQmx.AI.lvclass">)  [unwired: 7 in]
                }
                n142 = Merge Errors(w389, w388) -> (w384:errorcluster)
                n143 = Build Array (concatenate)(w391, w390) -> (w385:refnum<class "DAQmx.lvclass">[])
                n144 = call "DAQmx_SyncAll.vi"("error in (no error)"=w384, "Array in"=w385) -> ("error out"=w387:errorcluster, "Array out"=w386:refnum<class "DAQmx.lvclass">[])  [unwired: 8 in]
              }
              frame True {
                n145 = for {
                  tunnel: w413 -> [w422] mode=indexing
                  tunnel: [w421] -> w412 mode=indexing
                  shift-right: [w420] -> w410
                  shift-left: w406 -> [w419]
                  n146 = call "createDAQ.vi"("error in (no error)"=w419, "DAQ.Config"=w422) -> ("error out"=w420:errorcluster, "DAQ out"=w421:refnum<class "DAQ.lvclass">)  [unwired: 8 in]
                }
                n147 = for {
                  tunnel: w414 -> [w418] mode=indexing
                  tunnel: [w417] -> w411 mode=indexing
                  shift-right: [w416] -> w409
                  shift-left: w406 -> [w415]
                  n148 = call "createDAQ.vi"("error in (no error)"=w415, "DAQ.Config"=w418) -> ("error out"=w416:errorcluster, "DAQ out"=w417:refnum<class "DAQ.lvclass">)  [unwired: 8 in]
                }
                n149 = Build Array (concatenate)(w412, w411) -> (w408:refnum<class "DAQ.lvclass">[])
                n150 = Merge Errors(w410, w409) -> (w407:errorcluster)
              }
            }
            n151 = for {
              tunnel: [w380] -> w365 mode=indexing
              tunnel: w363 -> [w382] mode=indexing
              tunnel: [w381] -> w364 mode=indexing
              n152 = call <vilib>:"GetState.vi"("SMO"=w382) -> ("error out"=w378:errorcluster, "SMO State"=w380:T1, "SMO out"=w379:refnum<class "DAQ.lvclass">)  [unwired: 8 in]
              n153 = call <vilib>:"GetName.vi"("error in (no error)"=w378, "SMO"=w379) -> ("Name"=w381:string)  [unwired: 6 in, 3 out]
            }
            "Array 2" <- w364
            n154 = local write "Array"(w365) -> ()
            n155 = Bundle By Name(cluster=w366, "DAQ"=w363) -> (w374:T18)
            n156 = call <vilib>:"Add State(s) to Queue__jki_lib_state_machine.vi"("State(s) in (\"\")"=w377) -> ("States Out"=w376:string)  [unwired: 14 in]
          }
          frame "DAQ: start SMO" {
            # "reverse array so that master is started last"
            n157 = Unbundle By Name(w428) -> ("DAQ"=w425:refnum<class "DAQ.lvclass">[])
            n158 = Reverse 1D Array(array=w425) -> (reversed array=w427:refnum<class "DAQ.lvclass">[])
            n159 = for {
              shift-right: [w437] -> w426
              shift-left: w429 -> [w438]
              tunnel: w427 -> [w439] mode=indexing
              n160 = call <vilib>:"Start.vi"("error in (no error)"=w438, "SMO"=w439) -> ("error out"=w437:errorcluster)  [unwired: 8 in, 1 out]
            }
            n161 = for {
              tunnel: w425 -> [w435] mode=indexing
              shift-right: [w434] -> w423
              shift-left: w426 -> [w436]
              tunnel: [w433] -> w424 mode=indexing
              n162 = call <vilib>:"GetState.vi"("error in (no error)"=w436, "SMO"=w435) -> ("error out"=w434:errorcluster, "SMO State"=w433:T1)  [unwired: 7 in, 1 out]
            }
            n163 = local write "Array"(w424) -> ()
            n164 = call <vilib>:"Add State(s) to Queue__jki_lib_state_machine.vi"("State(s) in (\"\")"=w432) -> ("States Out"=w431:string)  [unwired: 14 in]
          }
          frame "DAQ: stop SMO" {
            n165 = Unbundle By Name(w445) -> ("DAQ"=w441:refnum<class "DAQ.lvclass">[])
            n166 = for {
              tunnel: w441 -> [w453] mode=indexing
              tunnel: w440 -> [w454]
              tunnel: [w450] -> w444 mode=indexing
              tunnel: [w449] -> w442 mode=indexing
              n167 = call <vilib>:"Stop.vi"("error in (no error)"=w454, "SMO"=w453) -> ("error out"=w452:errorcluster, "SMO out"=w451:refnum<class "DAQ.lvclass">)  [unwired: 8 in]
              n168 = call <vilib>:"GetState.vi"("error in (no error)"=w452, "SMO"=w451) -> ("error out"=w450:errorcluster, "SMO State"=w449:T1)  [unwired: 7 in, 1 out]
            }
            "Array" <- w442
            n169 = Merge Errors(w444) -> (w443:errorcluster)
            n170 = call <vilib>:"Add State(s) to Queue__jki_lib_state_machine.vi"("State(s) in (\"\")"=w448) -> ("States Out"=w447:string)  [unwired: 14 in]
          }
          frame "DAQ: destroy SMO" {
            n171 = Unbundle By Name(w459) -> ("DAQ"=w456:refnum<class "DAQ.lvclass">[])
            n172 = for {
              tunnel: [w468] -> w458 mode=indexing
              tunnel: w456 -> [w467] mode=indexing
              tunnel: w455 -> [w466]
              n173 = call <vilib>:"isStateMachineObject.vi"("error in (no error)"=w466, "SMO"=w467) -> ("error out"=w463:errorcluster, "is SMO?"=w465:bool, "SMO out"=w464:refnum<class "DAQ.lvclass">)  [unwired: 7 in]
              n174 = case shown="False" w465 {
                tunnel: [w469 w472] -> w468
                tunnel: w464 -> [_ w471]
                tunnel: w463 -> [w469 w470]
                frame False {
                }
                frame True {
                  n175 = call <vilib>:"Destroy.vi"("error in (no error)"=w470, "SMO"=w471) -> ("error out"=w472:errorcluster)  [unwired: 9 in]
                }
              }
            }
            n176 = Merge Errors(w458) -> (w457:errorcluster)
            n177 = call <vilib>:"Add State(s) to Queue__jki_lib_state_machine.vi"("State(s) in (\"\")"=w462) -> ("States Out"=w461:string)  [unwired: 14 in]
          }
          frame "DAQ: update config" {
            n178 = disable-structure shown="Enabled" {
              frame Disabled {
                n179 = Bundle By Name("DAQ.Config (AO)"="DAQ.Config (AO)", "DAQ.Config (AI)"="DAQ.Config (AI)", "DAQmx.AO.Config"="DAQmx.AO.config", "DAQmx.AI.Config"="DAQmx.AI.config") -> ()  [unwired: 1 in, 1 out]
              }
              frame Enabled {
              }
            }
            n180 = call <vilib>:"Add State(s) to Queue__jki_lib_state_machine.vi"("State(s) in (\"\")"=w476) -> ("States Out"=w475:string)  [unwired: 14 in]
          }
          frame "DAQ: setWaveform" {
            # "concatenate channels and send to DAQ SMOs"
            # "figure out which are AO channels"
            n181 = Unbundle By Name(w488) -> ("DAQ"=w482:refnum<class "DAQ.lvclass">[], "setWaveform"=w483:T17)
            n182 = call "DAQ_Manager.getAO_chan_and_sampling.vi"("error in (no error)"=w484, "DAQ"=w482) -> ("error out"=w486:errorcluster, "DAQ (AO)"=w487:refnum<class "DAQ.lvclass">[])  [unwired: 6 in, 2 out]
            n183 = call "Concatenate_and_SetWaveforms.vi"("error in (no error)"=w486, "AO Array"=w483, "DAQ (AO)"=w487) -> ("error out"=w485:errorcluster)  [unwired: 6 in, 2 out]
            n184 = call <vilib>:"Add State(s) to Queue__jki_lib_state_machine.vi"("State(s) in (\"\")"=w491) -> ("States Out"=w490:string)  [unwired: 14 in]
          }
        }
      }
    }
    frame Error {
    }
  }
  n185 = call-parent "Process.vi"("error in"=w9, "SMO"=w8) -> ("error out"=w6:errorcluster, "SMO out"=→"DAQ_Manager out":refnum<class "DAQ_Manager.lvclass">)  [unwired: 8 in]
  n186 = Merge Errors(w6, w5) -> (→"error out":errorcluster)
